vi "Select Analog Trigger Mode.vi"(8 "error in (no error)":errorcluster, 9 "Mode":enum16{"Edge", "Pulse", "Window", "Off"}(ring), 10 "Function":u16(ring) items=["Voltage: DC", "Voltage: AC", "Current: DC", "Current: AC", "2W Resistance", "4W Resistance", "Diode", "Capacitance", "Temperature", "Continuity", "Frequency", "Period", "Ratio", "Digitize Voltage", "Digitize Current"], 11 "VISA resource name":refnum<visa-resource-name>) -> (0 "error out":errorcluster, 3 "VISA resource name out":refnum<visa-resource-name>)   [LabVIEW 2009, in "Keithley DMM7510.lvlib"]
doc: "This VI sets the the mode of the analog trigger. Edge, Pulse/Width, Window or Off."
uses:
  Keithley DMM7510.lvlib
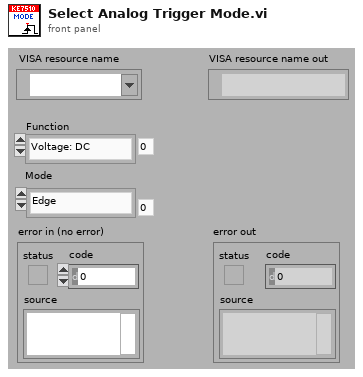
[diagram p1: front panel]
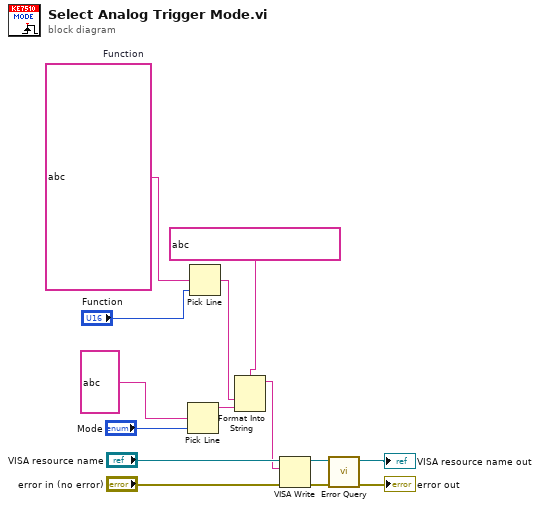
[diagram p0: block diagram]
diagram:
  w5 = string ?  # Function
  n1 = Pick Line(multi-line string=string ?, line index="Mode") -> (output string=w2:string)  [unwired: 1 in]
  n2 = Pick Line(multi-line string=w5, line index="Function") -> (output string=w3:string)  [unwired: 1 in]
  n3 = Format Into String(format string=string ?, w3, w2) -> (resulting string=w1:string)  [unwired: 2 in, 1 out]
  n4 = VISA Write(VISA resource name="VISA resource name", write buffer=w1, error in (no error)="error in (no error)") -> (VISA resource name out=w12:refnum<visa-resource-name>, error out=w9:errorcluster)  [unwired: 1 out]
  n5 = call "Error Query.vi"("error in (no error)"=w9, "VISA resource name"=w12) -> ("error out"=→"error out":errorcluster, "VISA resource name out"=→"VISA resource name out":refnum<visa-resource-name>)  [unwired: 6 in, 2 out]
